vi "Data Process Volt.vi"(8 "error in":errorcluster, 10 "Data Process.Volt":dbl[](array[numeric])) -> (0 "error out":errorcluster)   [LabVIEW 2020, in "Hardware DAQ.lvlib"]
doc: "Data Process Volt broadcast\n\n_____\nCreated using DQMH Event Scripter 6.1.0.128."
uses:
  Hardware DAQ.lvlib
  Data Process Volt Argument--cluster.ctl
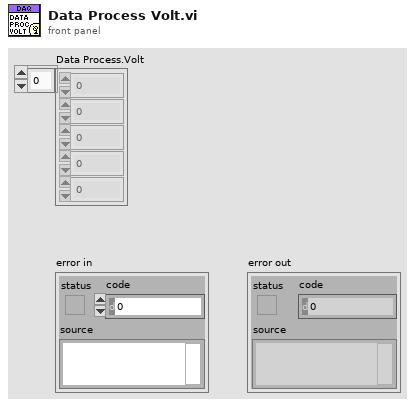
[diagram p1: front panel]
types:
  T1 = typedef "Hardware DAQ.lvlib/Data Process Volt Argument--cluster.ctl" = cluster{"Data Process.Volt":dbl[]}
  T2 = typedef "Hardware DAQ.lvlib/Broadcast Events--cluster.ctl" = cluster{"Module Did Init":refnum<user-event>, "Status Updated":refnum<user-event>, "Error Reported":refnum<user-event>, "Module Did Stop":refnum<user-event>, "Update Module Execution Status":refnum<user-event>, "Hardware Connected":refnum<user-event>, "Data Process Volt":refnum<user-event>, "Coil values":refnum<user-event>}
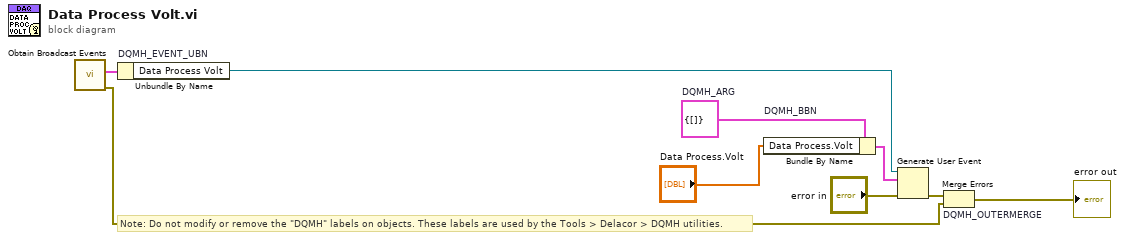
[diagram p0: block diagram]
diagram:
  w4 = T1 {"Data Process.Volt"=[]}  # DQMH_ARG
  # "Note: Do not modify or remove the \"DQMH\" labels on objects. These labels are used by the Tools > Delacor > DQMH utilities."
  n1 = call "Obtain Broadcast Events.vi"() -> ("error out"=w2:errorcluster, "Hardware DAQ Broadcast Events"=w1:T2)  [unwired: 10 in]
  n2 = Unbundle By Name "DQMH_EVENT_UBN"(w1) -> ("Data Process Volt"=w6:refnum<user-event>)
  n3 = Bundle By Name "DQMH_BBN"(cluster=w4, "Data Process.Volt"="Data Process.Volt") -> (w7:T1)
  n4 = Generate User Event(user event=w6, event data cluster=w7, error in="error in") -> (error out=w5:errorcluster)  [unwired: 1 in, 1 out]
  n5 = Merge Errors "DQMH_OUTERMERGE"(w5, w2) -> (→"error out":errorcluster)
